vi "DAQmx Create Channel (AI-Current-RMS).vi"(0 "task in":refnum<k21>, 1 "maximum value":dbl=0.01 format="%0.5f", 2 "minimum value":dbl=-0.01 format="%0.5f", 3 "input terminal configuration":i32(ring)=-1 items=["default"=-1, "RSE"=10083, "NRSE"=10078, "Differential"=10106, "Pseudodifferential"=12529], 5 "physical channels":tag, 7 "name to assign":string, 8 "external shunt resistor value":dbl=249.0 format="%0.2f", 9 "units":i32(ring)=10342 items=["Amps"=10342, "From Custom Scale"=10065], 11 "error in":errorcluster, 12 "custom scale name":tag, 14 "shunt resistor location":i32(ring)=-1 items=["default"=-1, "Internal"=10200, "External"=10167]) -> (4 "task out":refnum<k21>, 15 "error out":errorcluster)   [LabVIEW 2020]
doc: "Creates a channel to measure current RMS, the average (mean) power of the acquired current."
uses:
  nilvaiu.dll
panel:
  # "input limits"
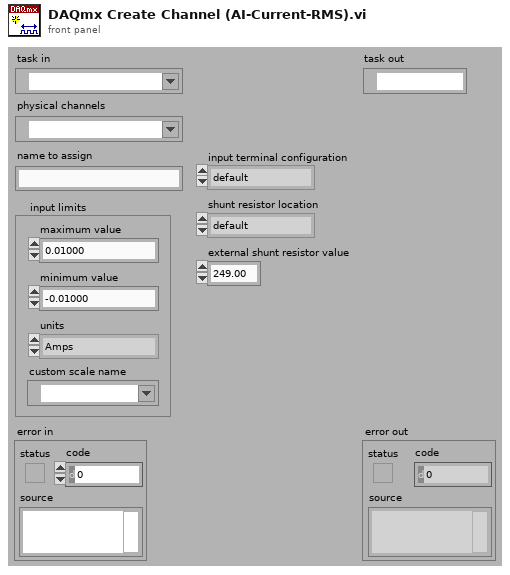
[diagram p1: front panel]
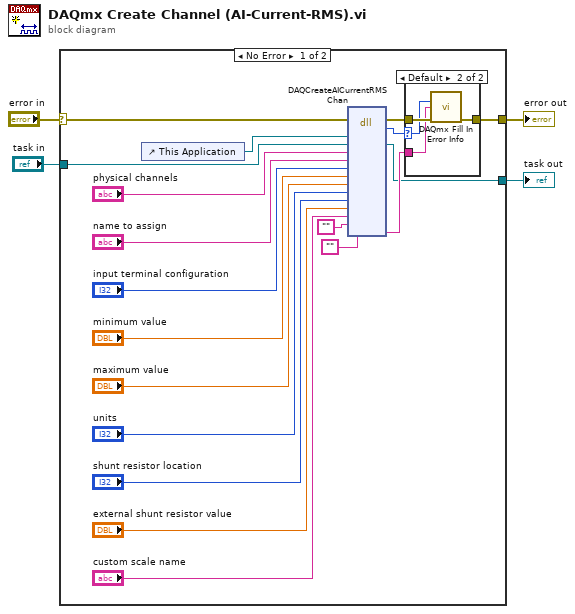
[diagram p0: block diagram]
diagram:
  n1 = case shown="No Error" "error in" {
    selector: "error in" -> [w17 w30]
    tunnel: [w18 w30] -> w4
    tunnel: [w16 w29] -> w3
    tunnel: "task in" -> [w15 w29]
    frame No Error {
      n2 = control-ref of="This Application"() -> (w20:refnum<vi>)
      n3 = dll-call lib="nilvaiu.*" fn="DAQCreateAICurrentRMSChan"(error in=w17, "lvAppRef"=w20, "refObjPtr"=w15, "physicalChannelName"="physical channels", "channelNameIn"="name to assign", "terminalConfig"="input terminal configuration", "minVal"="minimum value", "maxVal"="maximum value", "units"="units", "shuntResistorLoc"="shunt resistor location", "extShuntResistorVal"="external shunt resistor value", "customScaleName"="custom scale name", "channelNamesOut"="", "extendedErrorInfo"="") -> (error out=w23:errorcluster, "return type"=w22:i32, "refObjPtr"=w16:refnum<k21>, "extendedErrorInfo"=w21:string)  [unwired: 13 in, 1 out]
      n4 = case shown="Default" w22 {
        selector: w22 -> [_ w26]
        tunnel: w23 -> [w24 w28]
        tunnel: [w24 w27] -> w18
        tunnel: w21 -> [_ w25]
        frame 0 {
        }
        frame Default {
          n5 = call "DAQmx Fill In Error Info.vi"("status code"=w26, "extended error info"=w25, "error in"=w28) -> ("error out"=w27:errorcluster)  [unwired: 1 in, 11 out]
        }
      }
    }
    frame Error {
    }
  }
  "error out" <- w4
  "task out" <- w3
